vi "getComponentInfo.vi"(8 "error in (no error)":errorcluster, 11 "VGS_Project in":refnum<class "VGS_Project.lvclass">) -> (0 "error out":errorcluster, 2 "VGS_ComponentInfo out":refnum<class "VGS_ComponentInfo.lvclass">, 3 "VGS_Project out":refnum<class "VGS_Project.lvclass">)   [LabVIEW 2022 SP3, in "LV_VGS.lvlib" / "VGS_Project.lvclass"]
uses:
  VGS_Project.lvclass
  ComponentInfo/VGS_ComponentInfo.lvclass
  VGS_Project.lvclass/VGS_Project.ctl
  C:/Users/Andrey/Desktop/hajo/LV_VGS/vgs_project.dll
  vgs_project.dll
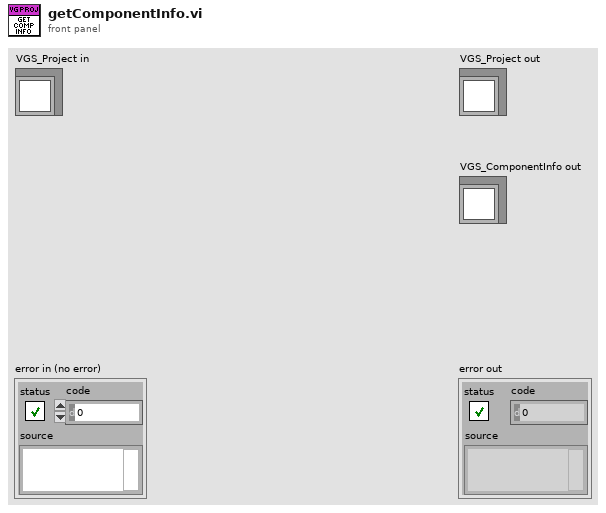
[diagram p1: front panel]
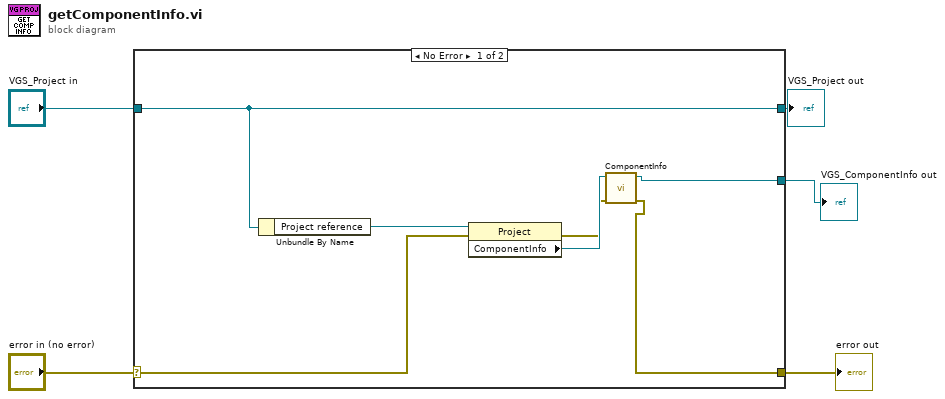
[diagram p0: block diagram]
diagram:
  n1 = case shown="No Error" "error in (no error)" {
    selector: "error in (no error)" -> [w10 w14]
    tunnel: [w6 w14] -> w2
    tunnel: [w12 w13] -> w3
    tunnel: "VGS_Project in" -> [w12 w13]
    tunnel: [w8 _] -> w1
    frame No Error {
      n2 = Unbundle By Name(w12) -> ("Project reference"=w11:refnum<k24>)
      n3 = property class="Project"(reference=w11, error in=w10) -> (error out=w7:errorcluster, "ComponentInfo"=w9:refnum<k24>)  [unwired: 1 out]
      n4 = call "ComponentInfo.vi"("error in (no error)"=w7, "new reference"=w9) -> ("error out"=w6:errorcluster, "VGS_ComponentInfo out"=w8:refnum<class "VGS_ComponentInfo.lvclass">)  [unwired: 8 in]
    }
    frame Error {
    }
  }
  "error out" <- w2
  "VGS_Project out" <- w3
  "VGS_ComponentInfo out" <- w1
